vi "Update Fields Table for Spartan 5.3.vi"(8 "error in (no error)":errorcluster, 11 "Connection Refnum":T1) -> (0 "error out":errorcluster, 3 "Connection Refnum":T1)   [LabVIEW 2011]
uses:
  SI.LIB/ODBC/SQL Controls/Connection Refnum.ctl
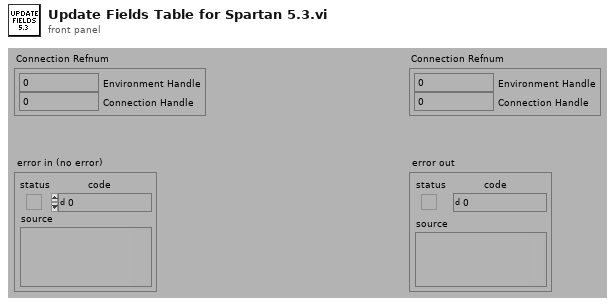
[diagram p1: front panel]
types:
  T1 = typedef "Connection Refnum.ctl" = cluster{"Environment Handle":i32, "Connection Handle":i32}
  T2 = typedef "Field Record.ctl" = cluster{"ixField":i32, "iSequenceOrder":i32, "sxFieldId":string, "sxSequenceId":string, "sDisplayName":string, "sValue":string, "sUnits":string, "nDataType":T3, "nNextItem":T4, "fSystem":bool, "fSystemValue":bool, "fRequired":bool, "fSetAtTest":bool, "fTestField":bool, "fDeleted":bool, "fIndexed":bool, "fFreeList":bool}
  T3 = typedef "Field DataTypes.ctl" = enum32{"text", "numeric", "list", "timestamp", "boolean"}
  T4 = typedef "Field NextItem.ctl" = enum32{"Reset", "Retain", "Auto-Increment"}
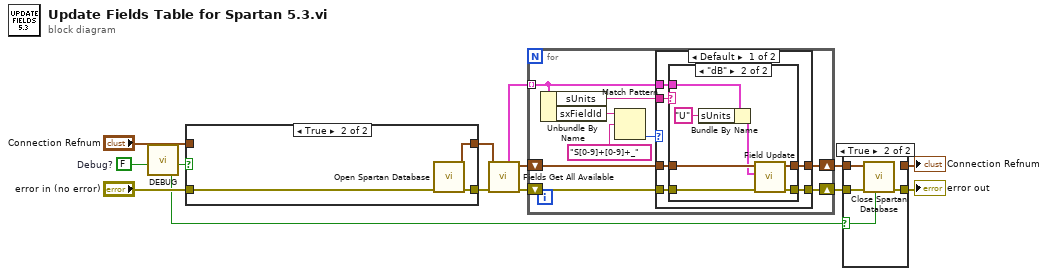
[diagram p0: block diagram]
diagram:
  w10 = FALSE  # Debug?
  n1 = call "DEBUG.vi"("Dev DEBUG? (f)"=w10) -> ("DEBUG?"=w8:bool)  [unwired: 1 in, 5 out]
  n2 = case shown="True" w8 {
    tunnel: "Connection Refnum" -> [w15 _]
    tunnel: "error in (no error)" -> [w14 w18]
    tunnel: [w14 w17] -> w6
    tunnel: [w15 w16] -> w7
    frame False {
    }
    frame True {
      n3 = call "Open Spartan Database.vi"("error in (no error)"=w18) -> ("error out"=w17:errorcluster, "Connection Refnum"=w16:T1)  [unwired: 2 in, 7 out]
    }
  }
  n4 = call "Fields Get All Available.vi"("error in (no error)"=w6, "Connection Refnum"=w7) -> ("error out"=w5:errorcluster, "Connection Refnum"=w3:T1, "Test Fields"=w4:T2[])  [unwired: 4 in, 3 out]
  n5 = for {
    shift-right: [w21] -> w2
    shift-left: w5 -> [w22]
    tunnel: w4 -> [w19] mode=indexing
    shift-right: [w23] -> w1
    shift-left: w3 -> [w24]
    n6 = Unbundle By Name(w19) -> ("sUnits"=w20:string, "sxFieldId"=w26:string)
    n7 = Match Pattern(string=w26, regular expression="S[0-9]+[0-9]+_") -> (offset past match=w25:i32)  [unwired: 1 in, 3 out]
    n8 = case shown="Default" w25 {
      tunnel: w24 -> [w32 w44]
      tunnel: [w31 w44] -> w23
      tunnel: w22 -> [w30 w43]
      tunnel: [w29 w43] -> w21
      tunnel: w20 -> [w33 _]
      tunnel: w19 -> [w28 _]
      frame Default {
        n9 = case shown="\"dB\"" w33 {
          tunnel: w32 -> [w35 w39]
          tunnel: [w35 w38] -> w31
          tunnel: w30 -> [w34 w40]
          tunnel: [w34 w37] -> w29
          tunnel: w28 -> [_ w42]
          frame Default {
          }
          frame "dB" {
            n10 = Bundle By Name(cluster=w42, "sUnits"="U") -> (w36:T2)
            n11 = call "Field Update.vi"("error in (no error)"=w40, "Field Record"=w36, "Connection Refnum"=w39) -> ("error out"=w37:errorcluster, "Connection Refnum"=w38:T1)  [unwired: 7 in]
          }
        }
      }
      frame -1 {
      }
    }
  }
  n12 = case shown="True" w8 {
    selector: w8 -> [_ w47]
    tunnel: w2 -> [w46 w50]
    tunnel: [w45 _] -> w9
    tunnel: [w46 w49] -> w11
    tunnel: w1 -> [w45 w48]
    frame False {
    }
    frame True {
      n13 = call "Close Spartan Database.vi"("Force Close? (f)"=w47, "error in (no error)"=w50, "Connection Refnum"=w48) -> ("error out"=w49:errorcluster)  [unwired: 2 in, 6 out]
    }
  }
  "Connection Refnum" <- w9
  "error out" <- w11
